vi "GetRidOf66.vi"(1 "error in (no error)":errorcluster) -> (0 "error out":errorcluster)   [LabVIEW 2018]
doc: "Removes timeout error"
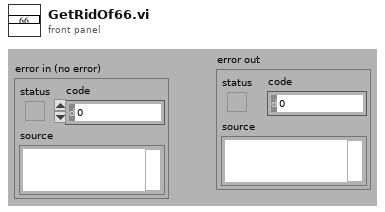
[diagram p1: front panel]
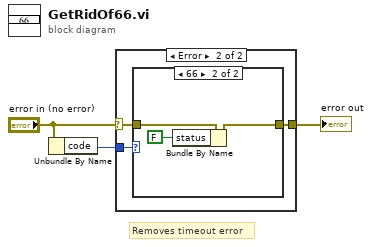
[diagram p0: block diagram]
diagram:
  # "Removes timeout error"
  n1 = Unbundle By Name("error in (no error)") -> ("code"=w1:i32)
  n2 = case shown="Error" "error in (no error)" {
    selector: "error in (no error)" -> [w4 w5]
    tunnel: [w4 w6] -> w3
    tunnel: w1 -> [_ w7]
    frame No Error {
    }
    frame Error {
      n3 = case shown="66" w7 {
        tunnel: [w8 w10] -> w6
        tunnel: w5 -> [w8 w11]
        frame Default {
        }
        frame 66 {
          n4 = Bundle By Name(cluster=w11, "status"=FALSE) -> (w10:errorcluster)
        }
      }
    }
  }
  "error out" <- w3
